vi "Find Item in Library.vi"(7 "Type":string, 8 "error in (no error)":errorcluster, 10 "Item Name":string, 11 "Library in":refnum<vi>) -> (0 "error out":errorcluster, 1 "Found ?":bool, 2 "ProjectItem out":refnum<vi>, 3 "Library out":refnum<vi>)   [LabVIEW 2019, in "Project Sync Tools.lvclass"]
uses:
  Project Sync Tools.lvclass
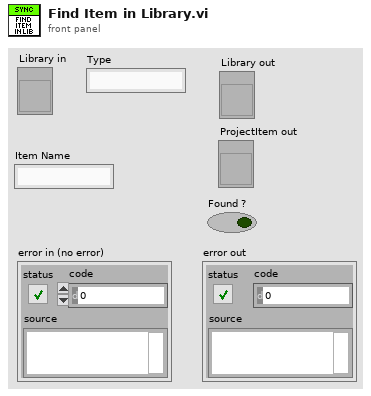
[diagram p1: front panel]
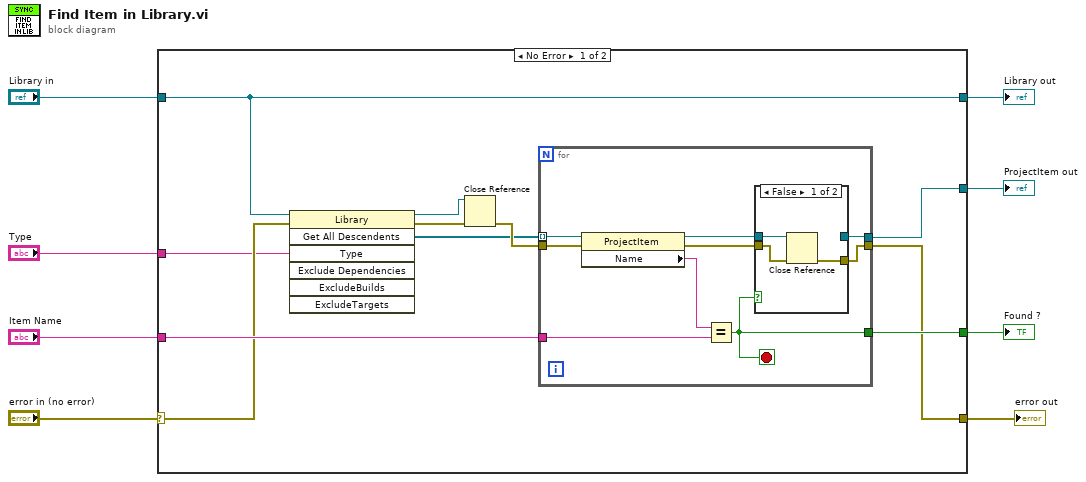
[diagram p0: block diagram]
diagram:
  n1 = case shown="No Error" "error in (no error)" {
    selector: "error in (no error)" -> [w11 w35]
    tunnel: [w16 _] -> w8
    tunnel: [w15 _] -> w7
    tunnel: "Item Name" -> [w13 _]
    tunnel: [w12 w35] -> w5
    tunnel: "Type" -> [w10 _]
    tunnel: "Library in" -> [w9 w34]
    tunnel: [w9 w34] -> w1
    frame No Error {
      n2 = invoke class="Library" method="Get All Descendents"(reference=w9, error in=w11, "Type"=w10) -> (reference out=w18:refnum<vi>, error out=w17:errorcluster, "All Descendents"=w14:refnum<vi>[])  [unwired: 4 in, 4 out]
      n3 = Close Reference(reference=w18, error in (no error)=w17) -> (error out=w19:errorcluster)
      n4 = for {
        tunnel: w14 -> [w28] mode=indexing
        tunnel: w13 -> [w27]
        tunnel: [w22] -> w12
        tunnel: [w25] -> w15
        tunnel: [w21] -> w16
        tunnel: w19 -> [w20]
        stop <- w25 stop-if-true
        n5 = property class="ProjectItem"(reference=w28, error in=w20) -> (reference out=w24:refnum<vi>, error out=w23:errorcluster, "Name"=w26:string)
        n6 = Equal?(x=w26, y=w27) -> (x = y?=w25:bool)
        n7 = case shown="False" w25 {
          tunnel: w24 -> [w31 w33]
          tunnel: w23 -> [w30 w32]
          tunnel: [w29 w32] -> w22
          tunnel: [_ w33] -> w21
          frame False {
            n8 = Close Reference(reference=w31, error in (no error)=w30) -> (error out=w29:errorcluster)
          }
          frame True {
          }
        }
      }
    }
    frame Error {
    }
  }
  "ProjectItem out" <- w8
  "Found ?" <- w7
  "error out" <- w5
  "Library out" <- w1
